vi "Init.vi"(8 "Error In":errorcluster, 10 "IConfigure":refnum<class "IConfigure.lvclass">, 11 "object in":refnum<class "OWON SDS1022.lvclass">) -> (0 "Error Out":errorcluster, 3 "object out":refnum<class "OWON SDS1022.lvclass">)   [LabVIEW 2023, in "OWON SDS1022.lvlib" / "OWON SDS1022.lvclass"]
uses:
  OWON SDS1022.lvclass
  OWON SDS1022.lvclass/OWON SDS1022.ctl
  HAL/Scope VISA/Scope VISA.lvclass
  HAL/Interfaces/IConfigure/IConfigure.lvclass
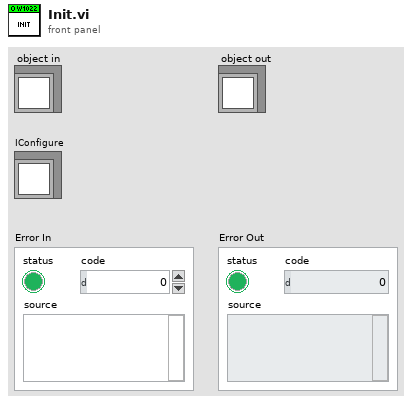
[diagram p1: front panel]
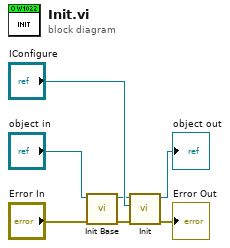
[diagram p0: block diagram]
diagram:
  n1 = call-dynamic "Init Base.vi"("Error In"="Error In", "object in"="object in") -> ("Error Out"=w6:errorcluster, "object out"=w2:refnum<class "OWON SDS1022.lvclass">)  [unwired: 8 in]
  n2 = call-parent "Init.vi"("Error In"=w6, "HAL.lvlib:IConfigure"="IConfigure", "object in"=w2) -> ("Error Out"=→"Error Out":errorcluster, "object out"=→"object out":refnum<class "OWON SDS1022.lvclass">)  [unwired: 7 in]
